vi "I2C Close.vi"(7 "I2C Channel":u8, 8 "Error In":errorcluster, 11 "LINX Device Config":T1) -> (0 "Error Out":errorcluster, 3 "LINX Device Config":T1)   [LabVIEW 2020, in "Device.lvlib"]
doc: "Close the specified I2C channel."
uses:
  Device.lvlib
  Type Defs/Error Type.ctl
  LMH-LINX.lvlib
  Type Defs/Interface.ctl
  Type Defs/Channels.ctl
  Type Defs/TCP Config.ctl
  Type Defs/LINX Device Config.ctl
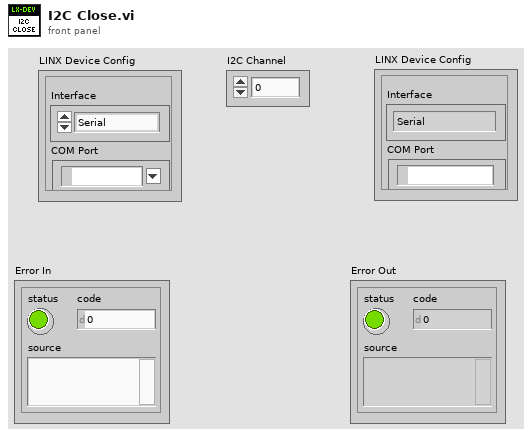
[diagram p1: front panel]
types:
  T1 = typedef "Device.lvlib/LINX Device Config.ctl" = cluster{"Interface":T2, "COM Port":refnum<visa-resource-name>, "TCP Configuration":T3, "Device Family":u8, "Device ID":u8, "Device Name":string, "TCP Ref":refnum<k5>, "Channels":T4}
  T2 = typedef "LMH-LINX.lvlib/Interface.ctl" = enum16{"Serial", "TCP"}
  T3 = typedef "Device.lvlib/TCP Config.ctl" = cluster{"IP Address":string, "Port":u16}
  T4 = typedef "LMH-LINX.lvlib/Channels.ctl" = cluster{"DI":u8[], "DO":u8[], "AI":u8[], "AO":u8[], "PWM":u8[], "QE":u8[], "UART":u8[], "I2C 2":u8[], "SPI":u8[], "CAN":u8[], "Servo":u8[], "AI Ref (V)":dbl, "AI Resolution (Bits)":u8, "AO Ref (V)":dbl, "AO Resolution (Bits)":u8}
  T5 = typedef "LMH-LINX.lvlib/Error Type.ctl" = enum16{"Unknown", "Timeout", "Corrupt Return Packet", "Unable To Connect", "Command Not Supported", "Channel DNE", "Invalid COM Config", "Firmware Version Mismatch", "myRIO Support", "CMD Specific Error", "Local IO Not Supported"}
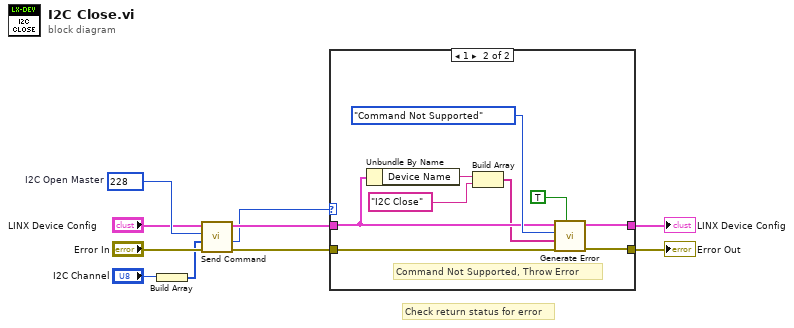
[diagram p0: block diagram]
diagram:
  w9 = u16 228  # I2C Open Master
  # "Check return status for error"
  n1 = Build Array("I2C Channel") -> (w2:u8[])
  n2 = call "Send Command.vi"("Error In"="Error In", "ARGS"=w2, "CMD"=w9, "LINX Device Config"="LINX Device Config") -> ("Error Out"=w4:errorcluster, "Status"=w1:u8, "LINX Device Config"=w6:T1)  [unwired: 4 in, 1 out]
  n3 = case shown="1" w1 {
    tunnel: [w12 w19] -> w7
    tunnel: w6 -> [w12 w15]
    tunnel: [w11 w20] -> w5
    tunnel: w4 -> [w11 w21]
    frame 0, Default {
      # "Status OK, No Data To Process"
    }
    frame 1 {
      # "Command Not Supported, Throw Error"
      n4 = Unbundle By Name(w15) -> ("Device Name"=w17:string)
      n5 = Build Array(w17, "I2C Close") -> (w14:string[])
      n6 = call "Generate Error.vi"("Is Warning? (False)"=TRUE, "Error In"=w21, "Arguments"=w14, "Error Type"=Error_Type."Command Not Supported", "LINX Device Config"=w15) -> ("Error Out"=w20:errorcluster, "Dup LINX Device Config"=w19:T1)  [unwired: 5 in]
    }
  }
  "Error Out" <- w5
  "LINX Device Config" <- w7
